vi "DAQmx Disconnect All Routing.vi"(0 "device in":tag, 11 "error in":errorcluster) -> (15 "error out":errorcluster)   [LabVIEW 2012]
doc: "Immediately aborts all active tasks associated with a device, disconnects any routes, and returns the device to an initialized state. Aborting a task immediately terminates the currently active operation, such as a read or a write. Aborting a task puts the task into an unstable but recoverable state. To recover the task, use DAQmx Start to restart the task or use DAQmx Stop to reset the task without starting it."
uses:
  <resource>/objmgr/daqmx.rc
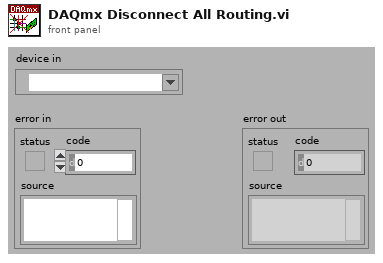
[diagram p1: front panel]
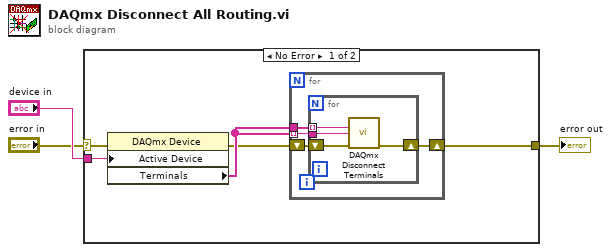
[diagram p0: block diagram]
diagram:
  n1 = case shown="No Error" "error in" {
    selector: "error in" -> [w6 w17]
    tunnel: "device in" -> [w8 _]
    tunnel: [w7 w17] -> w2
    frame No Error {
      n2 = property class="DAQmx Device"(error in=w6, "Active Device"=w8) -> (error out=w4:errorcluster, "Terminals"=w5:tag[])  [unwired: 1 in, 1 out]
      n3 = for {
        tunnel: w5 -> [w11] mode=indexing
        tunnel: w5 -> [w10]
        shift-right: [w12] -> w7
        shift-left: w4 -> [w9]
        n4 = for {
          tunnel: w11 -> [w13]
          shift-right: [w15] -> w12
          shift-left: w9 -> [w16]
          tunnel: w10 -> [w14] mode=indexing
          n5 = call <vilib>:"DAQmx Disconnect Terminals.vi"("source terminal"=w14, "destination terminal"=w13, "error in"=w16) -> ("error out"=w15:errorcluster)  [unwired: 12 in]
        }
      }
    }
    frame Error {
    }
  }
  "error out" <- w2
